vi "Year2019 Q3.vi"() -> ()   [LabVIEW 2018]
panel:
  out "Sum":dbl
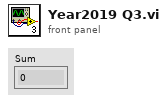
[diagram p1: front panel]
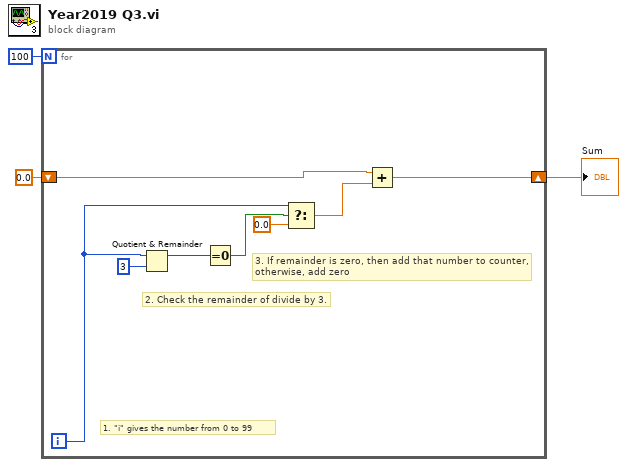
[diagram p0: block diagram]
diagram:
  n1 = for {
    N: 100 -> [_]
    shift-right: [w5] -> w2
    shift-left: 0.0 -> [w4]
    i -> [w7]
    # "1. \"i\" gives the number from 0 to 99"
    # "3. If remainder is zero, then add that number to counter,\notherwise, add zero"
    # "2. Check the remainder of divide by 3."
    n2 = Quotient & Remainder(x=w7, y=3) -> (x-y*floor(x/y)=w10:i32)  [unwired: 1 out]
    n3 = Equal To 0?(x=w10) -> (x = 0?=w9:bool)
    n4 = Select(t=w7, s=w9, f=0.0) -> (s? t:f=w6:dbl)
    n5 = Add(x=w4, y=w6) -> (x+y=w5:dbl)
  }
  "Sum" <- w2
